vi "Servo Read Angle.vi"(0 "Arduino Resource":T1={"VISA resource"="", "Board Type"=enum."Arduino Uno", "Connection Type"=enum."USB / Serial", "Bytes Per Packet (15)"=15}, 7 "Servo Number":u8=15, 11 "error in":errorcluster) -> (4 "Arduino Resource":T1={"VISA resource"="", "Board Type"=enum."Arduino Uno", "Connection Type"=enum."USB / Serial", "Bytes Per Packet (15)"=15}, 8 "Angle (Degrees)":u8=15, 15 "error out":errorcluster)   [LabVIEW 2011, in "LabVIEW Interface for Arduino.lvlib"]
doc: "Read the last angle in degrees written to the specified servo."
uses:
  LabVIEW Interface for Arduino.lvlib
  Private/Type Defs/Arduino Resource.ctl
  Private/Type Defs/Board Type.ctl
  Private/Type Defs/Command.ctl
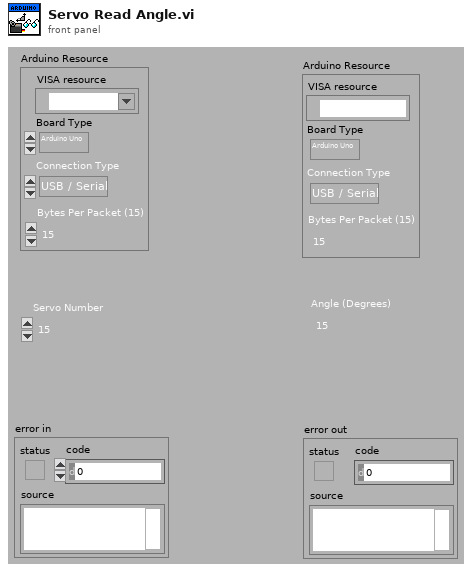
[diagram p1: front panel]
types:
  T1 = typedef "LabVIEW Interface for Arduino.lvlib/Arduino Resource.ctl" = cluster{"VISA resource":refnum<visa-resource-name>, "Board Type":T2, "Connection Type":enum8{"USB / Serial"}, "Bytes Per Packet (15)":u8}
  T2 = typedef "LabVIEW Interface for Arduino.lvlib/Board Type.ctl" = enum16{"Arduino Uno", "Dimuelanove w/Atmega 328", "Mega 2560", "Chipkit Uno32", "Chipkit Max32"}
  T3 = typedef "LabVIEW Interface for Arduino.lvlib/Command.ctl" = enum8{"setArduinoMode", "flushSerial", "setPinMode", "digitalWritePin", "digitalWritePort", "tone", "digitalReadPin", "digitalReadPort", "analogReadPin", "analogReadPort", "pwmWritePin", "pwmWritePort", "sevenSegment_Configure", "sevenSegment_Write", "I2C Init", "I2C Write", "I2C Read", "SPI Init", "SPI Set Bit Order", "SPI Set Clock Divider", "SPI Set Data Mode", "SPI Send / Receive", "SPI Close", "Servo Set Num Servos", "Servo Config Servo", "Servo Write Angle", "Servo Read Angle", "Servo Write Pulse Width", "Servo Read Pulse Width", "Servo Detach", "LCD Init", "LCD Set Size", "LCD Set Cursor Mode", "LCD Clear", "LCD Set Cursor Position", "LCD Print", "LCD Display Power", "LCD Scroll Display", "LCD Autoscroll", "LCD Print Direction", "LCD Create Custom Char", "LCD Print Custom Char", "contAcqOn", "contAcqOff", "getFirmwareVersion", "FiniteSampleStart"}
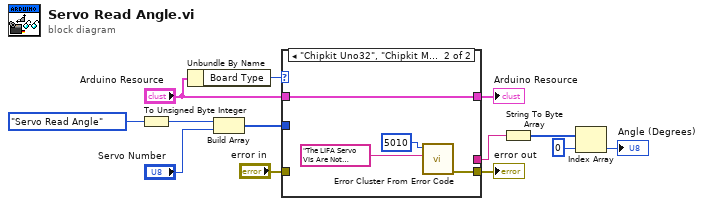
[diagram p0: block diagram]
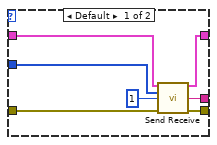
[diagram p2: hidden frame]
diagram:
  n1 = To Unsigned Byte Integer(number=Command."Servo Read Angle" ("Command")) -> (unsigned 8bit integer=w12:u8)
  n2 = Unbundle By Name("Arduino Resource") -> ("Board Type"=w1:T2)
  n3 = Build Array(w12, "Servo Number") -> (w6:u8[])
  n4 = case shown="\"Chipkit Uno32\", \"Chipkit Max32\"" w1 {
    tunnel: [w18 w22] -> w4
    tunnel: "Arduino Resource" -> [w19 w21]
    tunnel: w6 -> [w17 _]
    tunnel: "error in" -> [w16 _]
    tunnel: [w15 w21] -> w3
    tunnel: [w14 _] -> w2
    frame Default {
      n5 = call "Send Receive.vi"("Arduino Resource"=w19, "Data"=w17, "Bytes To Read (0)"=u8 1, "error in"=w16) -> ("Arduino Resource"=w15:T1, "Read Buffer"=w14:string, "error out"=w18:errorcluster)  [unwired: 9 in]
    }
    frame "Chipkit Uno32", "Chipkit Max32" {
      n6 = call <vilib>:"Error Cluster From Error Code.vi"("error message (\"\")"="The LIFA Servo VIs Are Not Supported On Chipkit Targets." ("source"), "error code (0)"=5010) -> ("error out"=w22:errorcluster)  [unwired: 7 in]
    }
  }
  "Arduino Resource" <- w3
  "error out" <- w4
  n7 = String To Byte Array(string=w2) -> (unsigned byte array=w11:u8[])
  n8 = Index Array(array=w11, index=0) -> (element=→"Angle (Degrees)":u8)
